vi "ep_Replace Range Utilization.vi"(8 "error in (no error)":errorcluster, 9 "system info in":refnum<class "EP System Info.lvclass">, 10 "full-range RMS values":dbl[](array[numeric]), 11 "waveforms in":waveform(dbl)[](array[waveform])) -> (0 "error out":errorcluster, 1 "system info out":refnum<class "EP System Info.lvclass">, 3 "actual ranges [%]":dbl[](array[numeric]))   [LabVIEW 2014, in "NI_EP_Power Quality.lvlib"]
uses:
  <vilib>/addons/Electrical Power/PQ/NI_EP_Power Quality.lvlib
  <vilib>/addons/Electrical Power/PQ/Common/Classes/System Info/EP System Info.lvclass
  <vilib>/Analysis/5stat.llb/RMS (DBL).vi
  <vilib>/Analysis/NI_AALPro.lvlib
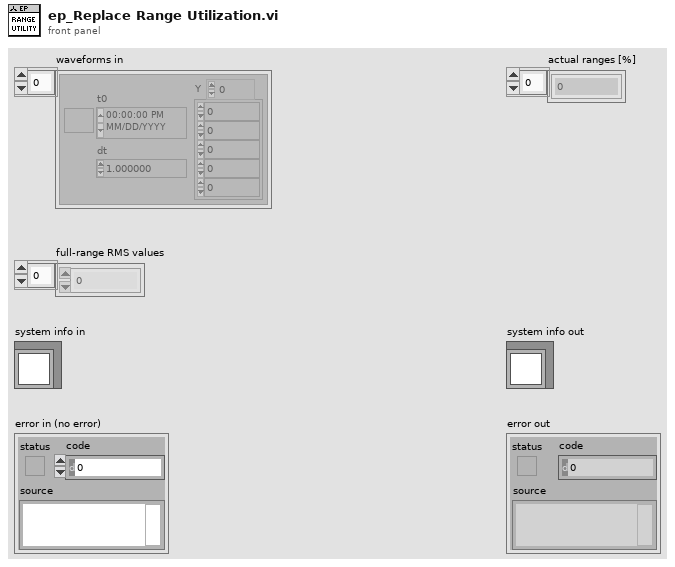
[diagram p1: front panel]
types:
  T1 = typedef "NI_EP_Power Quality.lvlib/ep_Channel Ranges.ctl" = cluster{"3-phase system ID":string, "ranges":dbl[]}
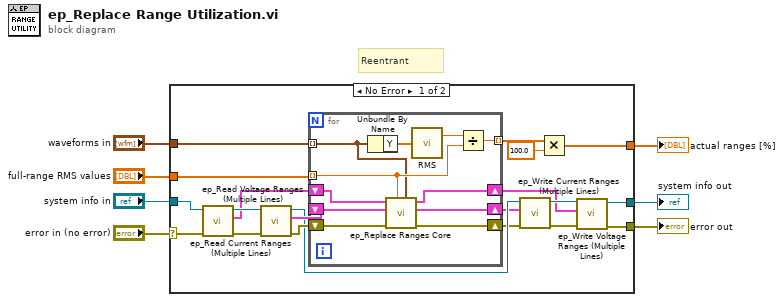
[diagram p0: block diagram]
diagram:
  # "Reentrant"
  n1 = case shown="No Error" "error in (no error)" {
    selector: "error in (no error)" -> [w20 w40]
    tunnel: "waveforms in" -> [w27 _]
    tunnel: "system info in" -> [w22 w39]
    tunnel: "full-range RMS values" -> [w26 _]
    tunnel: [w10 w39] -> w1
    tunnel: [w12 w40] -> w4
    tunnel: [w25 _] -> w2
    frame No Error {
      n2 = call <vilib>:"ep_Read Voltage Ranges (Multiple Lines).vi"("error in (no error)"=w20, "system info in"=w22) -> ("error out"=w19:errorcluster, "voltage ranges (multiline)"=w17:T1[], "system info out"=w21:refnum<class "EP System Info.lvclass">)  [unwired: 7 in]
      n3 = call <vilib>:"ep_Read Current Ranges (Multiple Lines).vi"("error in (no error)"=w19, "system info in"=w21) -> ("error out"=w16:errorcluster, "current ranges (multiline)"=w18:T1[], "system info out"=w15:refnum<class "EP System Info.lvclass">)  [unwired: 7 in]
      n4 = for {
        shift-right: [w38] -> w14
        shift-left: w16 -> [w30]
        tunnel: w27 -> [w34] mode=indexing
        tunnel: w26 -> [w35] mode=indexing
        tunnel: [w33] -> w24 mode=indexing
        shift-right: [w28] -> w9
        shift-left: w18 -> [w31]
        shift-right: [w29] -> w8
        shift-left: w17 -> [w32]
        n5 = Unbundle By Name(w34) -> ("Y"=w37:dbl[])
        n6 = call <vilib>:"ep_Replace Ranges Core.vi"("waveform"=w34, "full-range RMS values"=w35, "error in"=w30, "current ranges (multiline) in"=w31, "voltage ranges (multiline) in"=w32) -> ("error out"=w38:errorcluster, "current ranges (multiline) out"=w28:T1[], "voltage ranges (multiline) out"=w29:T1[])  [unwired: 4 in]
        n7 = call-poly <vilib>:"RMS.vi"("X"=w37) -> ("rms value"=w36:dbl)  [unwired: 1 out]
        n8 = Divide(x=w36, y=w35) -> (x/y=w33:dbl)
      }
      n9 = call <vilib>:"ep_Write Current Ranges (Multiple Lines).vi"("error in (no error)"=w14, "current ranges (multiline)"=w9, "system info in"=w15) -> ("error out"=w13:errorcluster, "system info out"=w11:refnum<class "EP System Info.lvclass">)  [unwired: 7 in]
      n10 = Multiply(x=w24, y=100.0) -> (x*y=w25:dbl[])
      n11 = call <vilib>:"ep_Write Voltage Ranges (Multiple Lines).vi"("error in (no error)"=w13, "voltage ranges (multiline)"=w8, "system info in"=w11) -> ("error out"=w12:errorcluster, "system info out"=w10:refnum<class "EP System Info.lvclass">)  [unwired: 7 in]
    }
    frame Error {
    }
  }
  "error out" <- w4
  "system info out" <- w1
  "actual ranges [%]" <- w2
